vi "libdaq_dac_set_wavepara.vi"(0 "error in (no error)":errorcluster, 1 "device_name":string, 2 "module_name":string, 7 "buf":dbl[](array[numeric])=[1.0], 9 "cycles":u32, 11 "frequency":dbl, 13 "trigger_mode":enum16{"AUTO", "SOFT", "HARD"}(ring)) -> (14 "error out":errorcluster, 15 "device_name":string, 16 "module_name":string)   [LabVIEW 2010, in "libdaqVI.lvlib"]
doc: "设置DAC模块的输出数据和工作模式"
uses:
  libdaqVI.lvlib
  dll/daqlib.dll
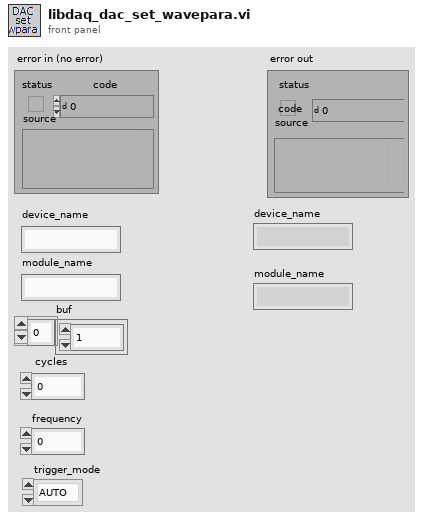
[diagram p1: front panel]
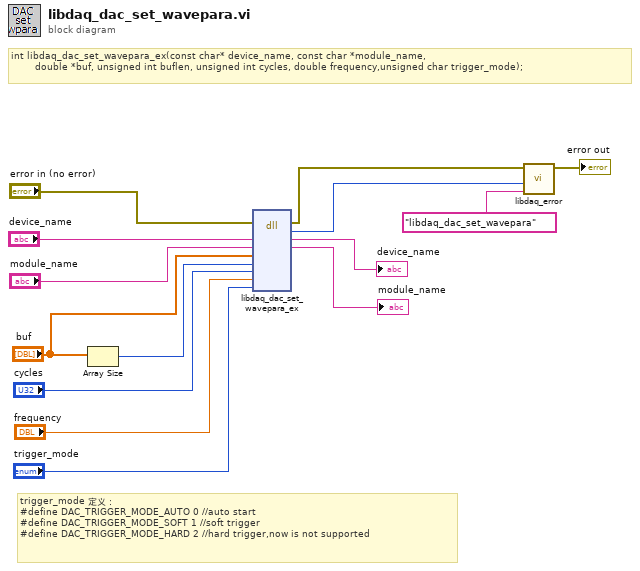
[diagram p0: block diagram]
diagram:
  # "trigger_mode 定义：\n#define DAC_TRIGGER_MODE_AUTO 0 //auto start\n#define DAC_TRIGGER_MODE_SOFT 1 //soft trigger\n#define DAC_TRIGGER_MODE_HARD 2 //hard trigger,now is not supported"
  # "int libdaq_dac_set_wavepara_ex(const char* device_name, const char *module_name,\n        double *buf, unsigned int buflen, unsigned int cycles, double frequency,unsigned char trigger_mode);"
  n1 = Array Size(array="buf") -> (size(s)=w5:i32)
  n2 = dll-call lib="E:/Product/Example/DAQ-USB3212/Labview/labview_2010/libdaqVI/dll/daqlib.dll" fn="libdaq_dac_set_wavepara_ex"(error in="error in (no error)", "device_name"="device_name", "module_name"="module_name", "buf"="buf", "buflen"=w5, "cycles"="cycles", "frequency"="frequency", "trigger_mode"="trigger_mode") -> (error out=w10:errorcluster, "return type"=w9:i32, "device_name"=→"device_name":string, "module_name"=→"module_name":string)  [unwired: 7 in, 1 out]
  n3 = call "libdaq_error.vi"("error source"="libdaq_dac_set_wavepara", "error code"=w9, "错误输入（无错误）"=w10) -> ("错误输出"=→"error out":errorcluster)  [unwired: 8 in]
